vi "Fetch Rx Data (U32).vi"(0 "niUsrpRio Session":T1={"Global Settings Register Bus"=refnum, "Radio 0 Settings Register Bus"=refnum, "Rx NI-USRP session"="", "Tx NI-USRP session"="", "FPGA Interface"=refnum, "RIO Interface Number"=0, "EEPROM Header"={"Checksum"=0, "Product Code"=0, "Hardware Current Version"=0, "Hardware Oldest Compatible Version"=0, "EEPROM Map Current Version"=0, "EEPROM Map Oldest Compatible Version"=0, "User Password"="", "Pointer to Factory Header"=0, "Pointer to User Header"=0, "Recommended Interval"=0, "Number of Reserved Bytes"=9, "Number of Daughterboards"=0, "Daughterboard IDs"=[], "Daughterboard Serial Numbers"=[]}, "Device Data Header"={"Checksum"=0, "Number of Channels"=0, "Number of Gain Settings"=[], "Pointer to Characterization Data"=[], "Number of Reserved Bytes"=27, "Number of Frequencies"=[]}, "EEPROM Characterization Header"={"Checksum"=0, "Date"=timestamp(0 s since 1904-01-01), "Temperature"=0.0, "Misc. Info"="", "Pointer to Device Data Header"=0, "Number of Reserved Bytes"=28}, "Characterization Data"=[], "Characterization Data Valid?"=FALSE, "Radio 1 Settings Register Bus"=refnum, "Radio Settings Bus Semaphore"=refnum} {"Characterization Data"."Frequencies [Hz]" format="%#_6p"; "EEPROM Characterization Header"."Pointer to Device Data Header" format="%x"; "EEPROM Characterization Header"."Checksum" format="%x"; "Device Data Header"."Pointer to Characterization Data" format="%x"; "Device Data Header"."Checksum" format="%x"; "EEPROM Header"."Pointer to User Header" format="%x"; "EEPROM Header"."Pointer to Factory Header" format="%x"; "EEPROM Header"."Product Code" format="%x"; "EEPROM Header"."Checksum" format="%x"}, 1 "scope":string, 2 "vertical range [Vpp]":dbl=2.0 format="%#_6p", 5 "number of samples":u32=8192, 9 "timeout":dbl=10.0 format="%#_gs", 11 "error in":errorcluster, 13 "leading samples to trim":u32) -> (3 "scaling (V/code)":dbl, 4 "niUsrpRio Session (out)":T1={"Global Settings Register Bus"=refnum, "Radio 0 Settings Register Bus"=refnum, "Rx NI-USRP session"="", "Tx NI-USRP session"="", "FPGA Interface"=refnum, "RIO Interface Number"=0, "EEPROM Header"={"Checksum"=0, "Product Code"=0, "Hardware Current Version"=0, "Hardware Oldest Compatible Version"=0, "EEPROM Map Current Version"=0, "EEPROM Map Oldest Compatible Version"=0, "User Password"="", "Pointer to Factory Header"=0, "Pointer to User Header"=0, "Recommended Interval"=0, "Number of Reserved Bytes"=9, "Number of Daughterboards"=0, "Daughterboard IDs"=[], "Daughterboard Serial Numbers"=[]}, "Device Data Header"={"Checksum"=0, "Number of Channels"=0, "Number of Gain Settings"=[], "Pointer to Characterization Data"=[], "Number of Reserved Bytes"=27, "Number of Frequencies"=[]}, "EEPROM Characterization Header"={"Checksum"=0, "Date"=timestamp(0 s since 1904-01-01), "Temperature"=0.0, "Misc. Info"="", "Pointer to Device Data Header"=0, "Number of Reserved Bytes"=28}, "Characterization Data"=[], "Characterization Data Valid?"=FALSE, "Radio 1 Settings Register Bus"=refnum, "Radio Settings Bus Semaphore"=refnum} {"Characterization Data"."Frequencies [Hz]" format="%#_6p"; "EEPROM Characterization Header"."Pointer to Device Data Header" format="%x"; "EEPROM Characterization Header"."Checksum" format="%x"; "Device Data Header"."Pointer to Characterization Data" format="%x"; "Device Data Header"."Checksum" format="%x"; "EEPROM Header"."Pointer to User Header" format="%x"; "EEPROM Header"."Pointer to Factory Header" format="%x"; "EEPROM Header"."Product Code" format="%x"; "EEPROM Header"."Checksum" format="%x"}, 6 "waveform data":u32[](array[numeric]), 15 "error out":errorcluster)   [LabVIEW 2013]
doc: "Fetches Rx data from the device. <b>Configure Stream</b> and <b>Initiate Stream</b> before calling this VI.\n\n<B>Input Parameters</B>\n\n<B>niUsrpRio Session</B> is the object created by the Open VI and used as the session handle for the USRP RIO design library.\n\n<B>scope</B> is the channel to fetch the data from. The options are \"rx/RF 0\", \"rx/RF 1\", \"tx/RF 0\", and \"tx/RF 1\".\n\n<B>vertical range</B> is the peak-to-peak range, in volts, of the acquired data. This control is used to accurately display the acquired data.\n\n<B>number of samples</B> to acquire.\n\n<B>timeout</B> is how long, in seconds, to keep retrying before giving up.\n\n<B>sample rate</B> the requested rate, in samples per second, that the signal will be sampled at. This control is used to accurately display the acquired data.\n\n<B>leading samples to trim</B> is the number of samples to throw away, starting from the first samples.\n\n<B>error in</B> describes error conditions that occur before this node runs. This input provides standard 'error in' functionality.\n\n<B>Output Parameters</B>\n\n<B>niUsrpRio Session (out)</B> is the niUsrpRio session used in all subsequent USRP RIO design library host VIs.\n\n<B>waveform data</B> contains the fetched data.\n\n<B>scaling</B> converts the waveform data into units of Volts.\n\n<B>error out</B> contains error information. This output provides standard 'error out' functionality."
uses:
  <instrlib>/niUsrpRio/Config/v1/Host/Public/niUsrpRio Session.ctl
  <instrlib>/_niInstr/Register Bus/v0/Host/Public/Register Bus Session.ctl
  <instrlib>/_niInstr/Register Bus/v0/Host/Private/Session Data.ctl
  <instrlib>/niUsrpRio/Config/v1/Host/Public/EEPROM Header.ctl
  <instrlib>/niUsrpRio/Config/v1/Host/Public/EEPROM Device Data Header.ctl
  <instrlib>/niUsrpRio/Config/v1/Host/Public/EEPROM Characterization Header.ctl
  <instrlib>/niUsrpRio/Config/v1/Host/Public/Characterization Data.ctl
  <instrlib>/niUsrpRio/Config/v1/Host/Public/IQ Imbalance.ctl
  Rx FPGA VI Reference.ctl
  <vilib>/rvi/interface/common/niFpgaWaitOnOcc.vi
  <vilib>/rvi/errors/niLvFpgaAdjustHostInterfaceError.vi
  <vilib>/rvi/interface/nirviMethod/nirviMethod.xnode
  <instrlib>/niUsrpRio/Config/v1/Host/niUsrpRio Config v1 Host.lvlib
  <vilib>/FPGAPlugInAG/Dynamic/niLvFpga_ReadFifo_Dynamic.vi
  <vilib>/rvi/errors/niLvFpgaMergeErrorWithErrorCode.vi
  <instrlib>/_niInstr/Register Bus/v0/Host/niInstr Register Bus v0 Host.lvlib
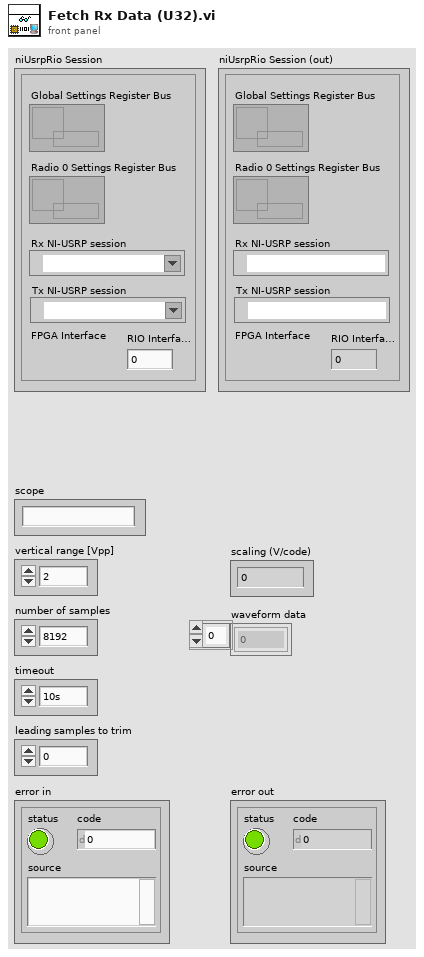
[diagram p1: front panel]
types:
  T1 = typedef "niUsrpRio Config v1 Host.lvlib/niUsrpRio Session.ctl" = cluster{"Global Settings Register Bus":T2, "Radio 0 Settings Register Bus":T2, "Rx NI-USRP session":refnum<k15>, "Tx NI-USRP session":refnum<k15>, "FPGA Interface":refnum<k20>, "RIO Interface Number":u32, "EEPROM Header":T3, "Device Data Header":T4, "EEPROM Characterization Header":T5, "Characterization Data":T6[], "Characterization Data Valid?":bool, "Radio 1 Settings Register Bus":T2, "Radio Settings Bus Semaphore":T8}
  T2 = typedef "niInstr Register Bus v0 Host.lvlib/Register Bus Session.ctl" = refnum<queue>
  T3 = typedef "niUsrpRio Config v1 Host.lvlib/EEPROM Header.ctl" = cluster{"Checksum":u32, "Product Code":u16, "Hardware Current Version":u16, "Hardware Oldest Compatible Version":u16, "EEPROM Map Current Version":u16, "EEPROM Map Oldest Compatible Version":u16, "User Password":string, "Pointer to Factory Header":u32, "Pointer to User Header":u32, "Recommended Interval":u16, "Number of Reserved Bytes":i32, "Number of Daughterboards":u8, "Daughterboard IDs":u16[], "Daughterboard Serial Numbers":string[]}
  T4 = typedef "niUsrpRio Config v1 Host.lvlib/EEPROM Device Data Header.ctl" = cluster{"Checksum":u32, "Number of Channels":u8, "Number of Gain Settings":u16[], "Pointer to Characterization Data":u32[], "Number of Reserved Bytes":i32, "Number of Frequencies":u16[]}
  T5 = typedef "niUsrpRio Config v1 Host.lvlib/EEPROM Characterization Header.ctl" = cluster{"Checksum":u32, "Date":timestamp, "Temperature":sgl, "Misc. Info":string, "Pointer to Device Data Header":u32, "Number of Reserved Bytes":i32}
  T6 = typedef "niUsrpRio Config v1 Host.lvlib/Characterization Data.ctl" = cluster{"Gains[dB]":dbl[], "Frequencies [Hz]":dbl[], "IQ Imbalance Table":T7[], "Measured Gains[dB]":dbl[][]}
  T7 = typedef "niUsrpRio Config v1 Host.lvlib/IQ Imbalance.ctl" = cluster{"Gain Imbalance [linear]":dbl, "Phase Imbalance [radians]":dbl, "Offset":cdb}
  T8 = typedef "Semaphore RefNum" = refnum<k1>
  T9 = typedef "Rx FPGA VI Reference.ctl" = refnum<k20>
  T10 = typedef "niUsrpRio Config v1 Host.lvlib/RF Channel.ctl" = enum16{"0", "1", "All"}
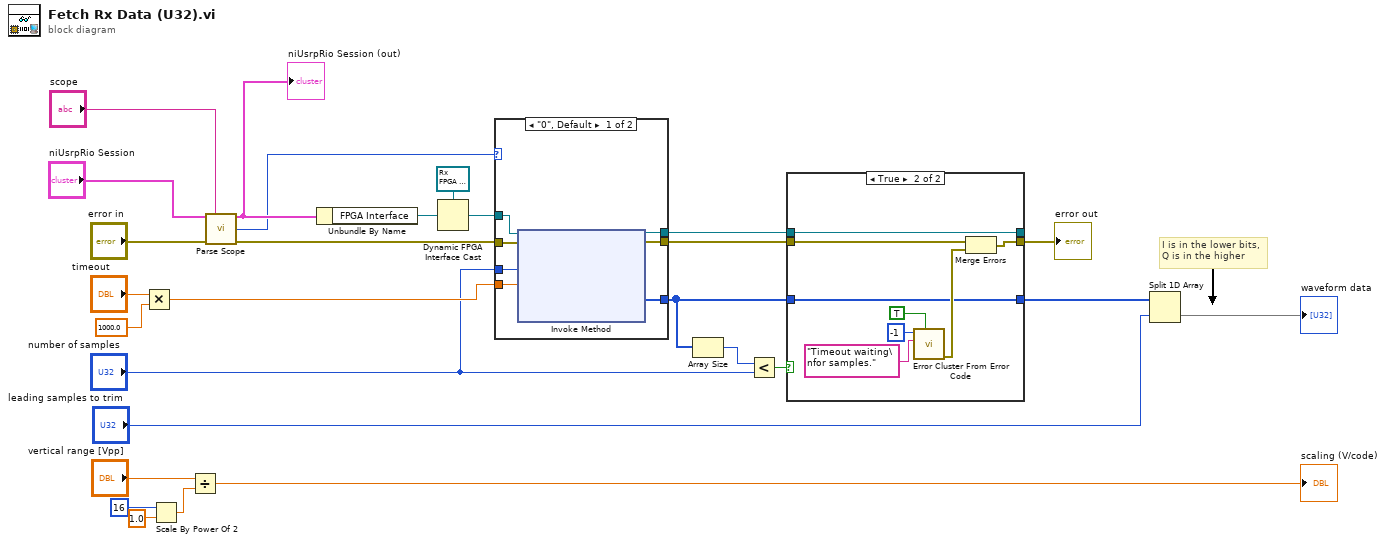
[diagram p0: block diagram]
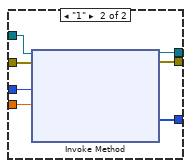
[diagram p2: hidden frame]
diagram:
  # "I is in the lower bits,\nQ is in the higher"
  n1 = Multiply(x="timeout", y=1000.0) -> (x*y=w22:dbl)
  n2 = Scale By Power Of 2(n=i16 16 ("ADC Resolution (bits)"), x=1.0) -> (x*2^n=w14:dbl)
  n3 = Divide(x="vertical range [Vpp]", y=w14) -> (x/y=→"scaling (V/code)":dbl)
  n4 = call <instrlib>:"Parse Scope.vi"("niUsrpRio Session"="niUsrpRio Session", "scope"="scope", "Error In"="error in") -> ("niUsrpRio Session (out)"=w5:T1, "Device Subfunction Channel"=w3:T10, "Error Out"=w7:errorcluster)  [unwired: 4 in, 6 out]
  "niUsrpRio Session (out)" <- w5
  n5 = Unbundle By Name(w5) -> ("FPGA Interface"=w4:refnum<k20>)
  n6 = Dynamic FPGA Interface Cast(Session In=T9 refnum ("Type"), Type=w4) -> (Session Out=w27:T9)
  n7 = case shown="\"0\", Default" w3 {
    tunnel: w27 -> [w34 w39]
    tunnel: [w33 w40] -> w26
    tunnel: [w32 w38] -> w25
    tunnel: w22 -> [w31 w35]
    tunnel: "number of samples" -> [w30 w36]
    tunnel: [w29 w37] -> w11
    tunnel: w7 -> [w28 w41]
    frame "0", Default {
      n8 = xnode "Invoke Method"("FPGA VI Reference In"=w34, "error in"=w28, "Number of Elements"=w30, "Timeout (ms)"=w31) -> ("FPGA VI Reference Out"=w32:T9, "error out"=w33:errorcluster, "Data"=w29:u32[])  [unwired: 1 out]
    }
    frame "1" {
      n9 = xnode "Invoke Method"("FPGA VI Reference In"=w39, "error in"=w41, "Number of Elements"=w36, "Timeout (ms)"=w35) -> ("FPGA VI Reference Out"=w38:T9, "error out"=w40:errorcluster, "Data"=w37:u32[])  [unwired: 1 out]
    }
  }
  n10 = Array Size(array=w11) -> (size(s)=w10:i32)
  n11 = Less?(x=w10, y="number of samples") -> (x < y?=w20:bool)
  n12 = case shown="True" w20 {
    tunnel: w25 -> [w44 w52]
    tunnel: w26 -> [w43 w49]
    tunnel: [w44 w52] -> _
    tunnel: [w43 w48] -> w18
    tunnel: [w42 w45] -> w9
    tunnel: w11 -> [w42 w45]
    frame False {
    }
    frame True {
      n13 = call <vilib>:"Error Cluster From Error Code.vi"("show call chain? (False)"=TRUE, "error message (\"\")"="Timeout waiting\nfor samples." ("error message (\"\")"), "error code (0)"=-1) -> ("error out"=w47:errorcluster)  [unwired: 6 in]
      n14 = Merge Errors(w49, w47) -> (w48:errorcluster)
    }
  }
  "error out" <- w18
  n15 = Split 1D Array(array=w9, index="leading samples to trim") -> (second subarray=→"waveform data":u32[])  [unwired: 1 out]
